vi "Create IO Control.vi"(8 "error in (no error)":errorcluster, 10 "IO Control":T2 {"Signals"."Response"."Byte Order" items=["Little Endian", "Big Endian"]; "Signals"."Response"."Data Type" items=["Signed", "Unsigned", "IEEE Float"]; "Signals"."Cmd"."Byte Order" items=["Little Endian", "Big Endian"]; "Signals"."Cmd"."Data Type" items=["Signed", "Unsigned", "IEEE Float"]}, 11 "Section Ptr":T1 format="%.0x") -> (0 "error out":errorcluster, 3 "Parent Ref out":T1 format="%.0x")   [LabVIEW 2015, in "Diagnostics Addon System Explorer.lvlib"]
uses:
  Diagnostics Addon System Explorer.lvlib
  Shared/Types/IO Control Parameters.ctl
  Shared/Types/Command Response Signals.ctl
  Shared/Types/Signal Parameters.ctl
  <vilib>/NI Veristand/Custom Device API/Custom Device Item Ref.ctl
  Types/FG Action.ctl
  Shared/Types/MessageType Selector.ctl
  <vilib>/NI Veristand/Custom Device API/NI VeriStand - Get Item Property.vi
  <vilib>/NI Veristand/Custom Device API/Get Item Property (U32).vi
  <vilib>/NI Veristand/Custom Device API/NI VeriStand - Set Item Property.vi
  <vilib>/NI Veristand/Custom Device API/Set Item Property (U32).vi
  Shared/SubVIs/GUID Lookup.vi
  <vilib>/NI Veristand/Custom Device API/Custom Device API.lvlib
  Shared/Diagnostics Addon Shared.lvlib
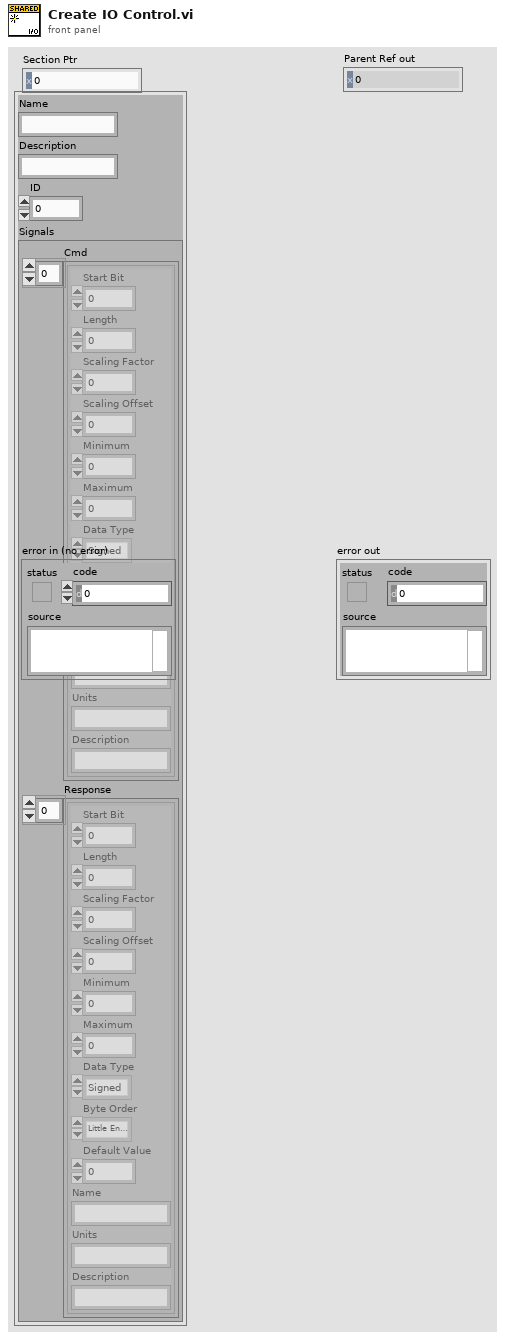
[diagram p1: front panel]
types:
  T1 = typedef "Custom Device API.lvlib/Custom Device Item Ref.ctl" = u64
  T2 = typedef "Diagnostics Addon Shared.lvlib/IO Control Parameters.ctl" = cluster{"Name":string, "Description":string, "ID":u16, "Signals":T3}
  T3 = typedef "Diagnostics Addon Shared.lvlib/Command Response Signals.ctl" = cluster{"Cmd":T4[], "Response":T4[]}
  T4 = typedef "Diagnostics Addon Shared.lvlib/Signal Parameters.ctl" = cluster{"Start Bit":u8, "Length":u8, "Scaling Factor":dbl, "Scaling Offset":dbl, "Minimum":dbl, "Maximum":dbl, "Data Type":u32, "Byte Order":u32, "Default Value":dbl, "Name":string, "Units":string, "Description":string}
  T5 = typedef "Diagnostics Addon Shared.lvlib/MessageType Selector.ctl" = enum16{"DID", "PID", "CPID", "Write Memory", "Read Memory", "DTC Control", "IO Cmd", "IO Resp", "Routine Start Cmd", "Routine Start Resp", "Routine Status Cmd", "Routine Status Resp", "Routine Stop Cmd", "Routine Stop Resp"}
  T6 = typedef "Diagnostics Addon System Explorer.lvlib/FG Action.ctl" = enum16{"Get", "Set"}
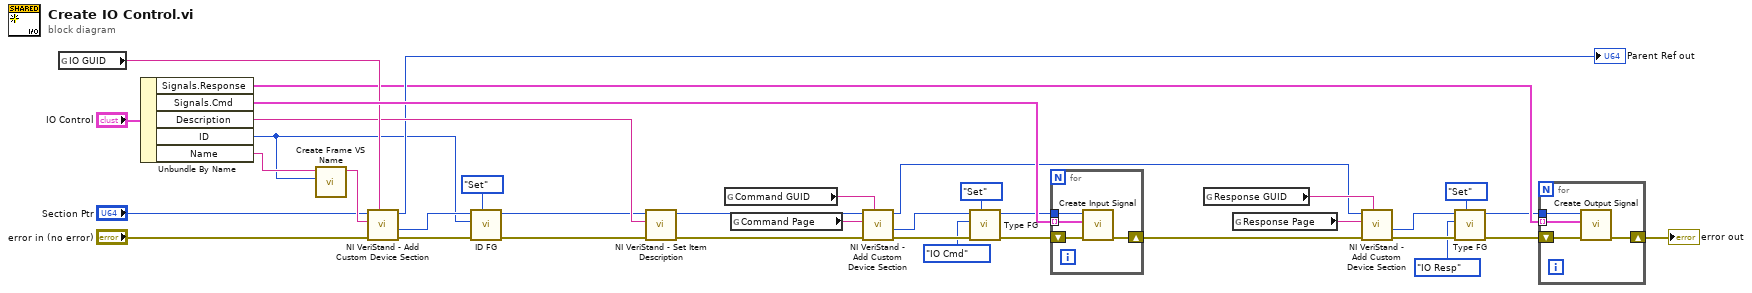
[diagram p0: block diagram]
diagram:
  n1 = global read "GUID Lookup.vi" "IO GUID"() -> (w33:string)
  n2 = Unbundle By Name("IO Control") -> ("Signals.Response"=w27:T4[], "Signals.Cmd"=w35:T4[], "Description"=w30:string, "ID"=w13:u16, "Name"=w16:string)
  n3 = call "Create Frame VS Name.vi"("PID Number"=w13, "PID Name"=w16) -> ("VS Name"=w36:string)  [unwired: 9 in]
  n4 = call <vilib>:"NI VeriStand - Add Custom Device Section.vi"("GUID (Default Section)"=w33, "error in (no error)"="error in (no error)", "Section Name"=w36, "Parent Ref in"="Section Ptr") -> ("error out"=w15:errorcluster, "Section Ptr"=w14:T1, "Parent Ref out"=→"Parent Ref out":T1)  [unwired: 4 in, 1 out]
  n5 = call "ID FG.vi"("Action"=FG_Action."Set", "error in (no error)"=w15, "ID"=w13, "Device Item Ref in"=w14) -> ("error out"=w11:errorcluster, "Device Item Ref out"=w10:T1)  [unwired: 5 in, 1 out]
  n6 = call <vilib>:"NI VeriStand - Set Item Description.vi"("error in (no error)"=w11, "Description"=w30, "Item Ref in"=w10) -> ("error out"=w21:errorcluster, "Item Ref out"=w20:T1)  [unwired: 6 in, 1 out]
  n7 = global read "GUID Lookup.vi" "Command GUID"() -> (w25:string)
  n8 = global read "GUID Lookup.vi" "Command Page"() -> (w26:string)
  n9 = call <vilib>:"NI VeriStand - Add Custom Device Section.vi"("GUID (Default Section)"=w25, "error in (no error)"=w21, "Section Name"=w26, "Parent Ref in"=w20) -> ("error out"=w8:errorcluster, "Section Ptr"=w18:T1, "Parent Ref out"=w22:T1)  [unwired: 4 in, 1 out]
  n10 = call "Type FG.vi"("Action"=FG_Action."Set", "error in (no error)"=w8, "Type"=MessageType_Selector."IO Cmd", "Device Item Ref in"=w18) -> ("error out"=w7:errorcluster, "Device Item Ref out"=w9:T1)  [unwired: 5 in, 1 out]
  n11 = for {
    shift-right: [w39] -> w19
    shift-left: w7 -> [w40]
    tunnel: w35 -> [w37] mode=indexing
    tunnel: w9 -> [w38]
    n12 = call "Create Input Signal.vi"("error in (no error)"=w40, "Signal Parameters"=w37, "Section Ptr"=w38) -> ("error out"=w39:errorcluster)  [unwired: 7 in, 1 out]
  }
  n13 = global read "GUID Lookup.vi" "Response GUID"() -> (w24:string)
  n14 = global read "GUID Lookup.vi" "Response Page"() -> (w23:string)
  n15 = call <vilib>:"NI VeriStand - Add Custom Device Section.vi"("GUID (Default Section)"=w24, "error in (no error)"=w19, "Section Name"=w23, "Parent Ref in"=w22) -> ("error out"=w4:errorcluster, "Section Ptr"=w17:T1)  [unwired: 4 in, 2 out]
  n16 = call "Type FG.vi"("Action"=FG_Action."Set", "error in (no error)"=w4, "Type"=MessageType_Selector."IO Resp") -> ("error out"=w3:errorcluster)  [unwired: 6 in, 2 out]
  n17 = for {
    shift-right: [w41] -> w28
    shift-left: w3 -> [w43]
    tunnel: w27 -> [w42] mode=indexing
    tunnel: w17 -> [w44]
    n18 = call "Create Output Signal.vi"("error in (no error)"=w43, "Signal Parameters"=w42, "Section Ptr"=w44) -> ("error out"=w41:errorcluster)  [unwired: 7 in, 1 out]
  }
  "error out" <- w28
